vi "RegisterDataPlugin.vi"(8 "error in":errorcluster, 11 "path":path) -> (0 "error out":errorcluster)   [LabVIEW 2020]
uses:
  <vilib>/Platform/storage/utility/Register DataPlugin by URI.vi
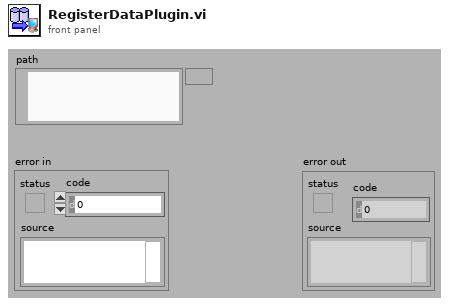
[diagram p1: front panel]
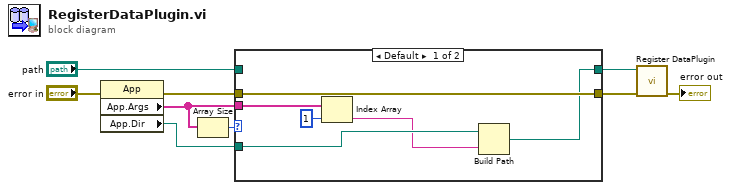
[diagram p0: block diagram]
diagram:
  n1 = property class="App"(error in="error in") -> (error out=w8:errorcluster, "App.Args"=w4:string[], "App.Dir"=w3:path)  [unwired: 1 in, 1 out]
  n2 = Array Size(array=w4) -> (size(s)=w9:i32)
  n3 = case shown="Default" w9 {
    tunnel: [w13 w17] -> w7
    tunnel: w8 -> [w13 w17]
    tunnel: "path" -> [_ w16]
    tunnel: [w10 w16] -> w5
    tunnel: w4 -> [w15 _]
    tunnel: w3 -> [w12 _]
    frame Default {
      n4 = Index Array(array=w15, index=1) -> (element=w11:string)
      n5 = Build Path(base path=w12, name or relative path=w11) -> (appended path=w10:path)
    }
    frame 1 {
    }
  }
  n6 = call-poly <vilib>:"Register DataPlugin.vi"("error in (no error)"=w7, "DataPlugin URI path (*.uri)"=w5) -> ("error out"=→"error out":errorcluster)  [unwired: 7 in, 2 out]
